vi "PDF_Interface_PDF Protokoll Dichtheitstest.vi"(8 "error in (no error)":errorcluster caption="Fehler (Eingang, kein Fehler)", 11 "Save PDF File Path":path) -> (0 "error out":errorcluster caption="Fehler (Ausgang)")   [LabVIEW 2020, in "Erweiterte Konfig.lvlib"]
uses:
  Erweiterte Konfig.lvlib
  Dichtheitstest Umfang.ctl
  Sprachverwaltung/FGV Aktion Tabelle zerlegen.ctl
  System Einstellungen V2/Aktioen FGV System Konstanten.ctl
  Status Dichtheitstest Aktionen.ctl
  FGV PID Aktionen.ctl
  PDF_Interface/PDF Protokoll Standard Kopf Optionen.ctl
  <vilib>/Simplicity AI/SAI_PDF_API/Classes/Context/Controls/SAI_PDF_PDF Details.ctl
  PDF_Interface/PDF Interface Helper/PDFContentType.ctl
  PDF_Interface/PDF Interface Helper/PDFTableContentType.ctl
  PDF_Interface/PDF Interface Helper/PDFResults.ctl
  PDF_Interface/PDF Interface Helper/PDFResultPictures.ctl
  PDF_Interface/PDF Interface Helper/PDFCommentPosition.ctl
  PDF_Interface/PDF Interface Helper/PDFPageBreak.ctl
  PDF_Interface/PDF Interface Helper/PDFTablePictures.ctl
  PDF_Interface/PDF Interface Helper/PDFBemerkung.ctl
  <vilib>/Simplicity AI/SAI_PDF_API/Classes/Context/Controls/SAI_PDF_Text Align.ctl
  <vilib>/Simplicity AI/SAI_PDF_API/Classes/Context/Controls/SAI_PDF_Font.ctl
  <vilib>/Simplicity AI/SAI_PDF_API/Classes/Context/Controls/SAI_PDF_Font Encoding.ctl
  Allgemein/allgemeine Sub-VIs.lvlib
  System Einstellungen V2/System Einstellungen V2.lvlib
  Sprachverwaltung/Sprachverwaltung.lvlib
  PDF_Interface/PDF Interface.lvlib
  <vilib>/Simplicity AI/SAI_PDF_API/Classes/Context/Context.lvclass
  PDF_Interface/PDF Interface Helper/PDF Interface Helper.lvlib
  Linearisierung V2/Protokoll/Protokoll.lvlib
panel:
  out "Dichtheitstest Umfang":T1 items=["Pumpe / Filter / FT-IR / PNS", "Pumpe / Filter / FT-IR", "Filter / FT-IR", "FT-IR"]
  out "zul. Druckabfall:":string
  out "Dauer Dichtheitstest:":string
  out "Bestanden":bool caption="Boolesch"
  out "Druckanstieg:":string
  out "Enddruck:":string
  out "Startdruck:":string
  out "Umfang:":string
  out "Endzeit:":string
  out "Startzeit:":string
  out "Ser.Nr.:":string caption="Serien Nummer:"
  out "Messgerät:":string
  # "Dichtheitstest"
  # "mbar"
  # "mbar"
  # "mbar"
  # "IAG-Industrie Automatisierungsgeschellschaft m.b.H.    l  Industriestraße 2    l    2722Weikersdorf     )+43262221734 7+43262221734655"
  # "mbar"
  # "s"
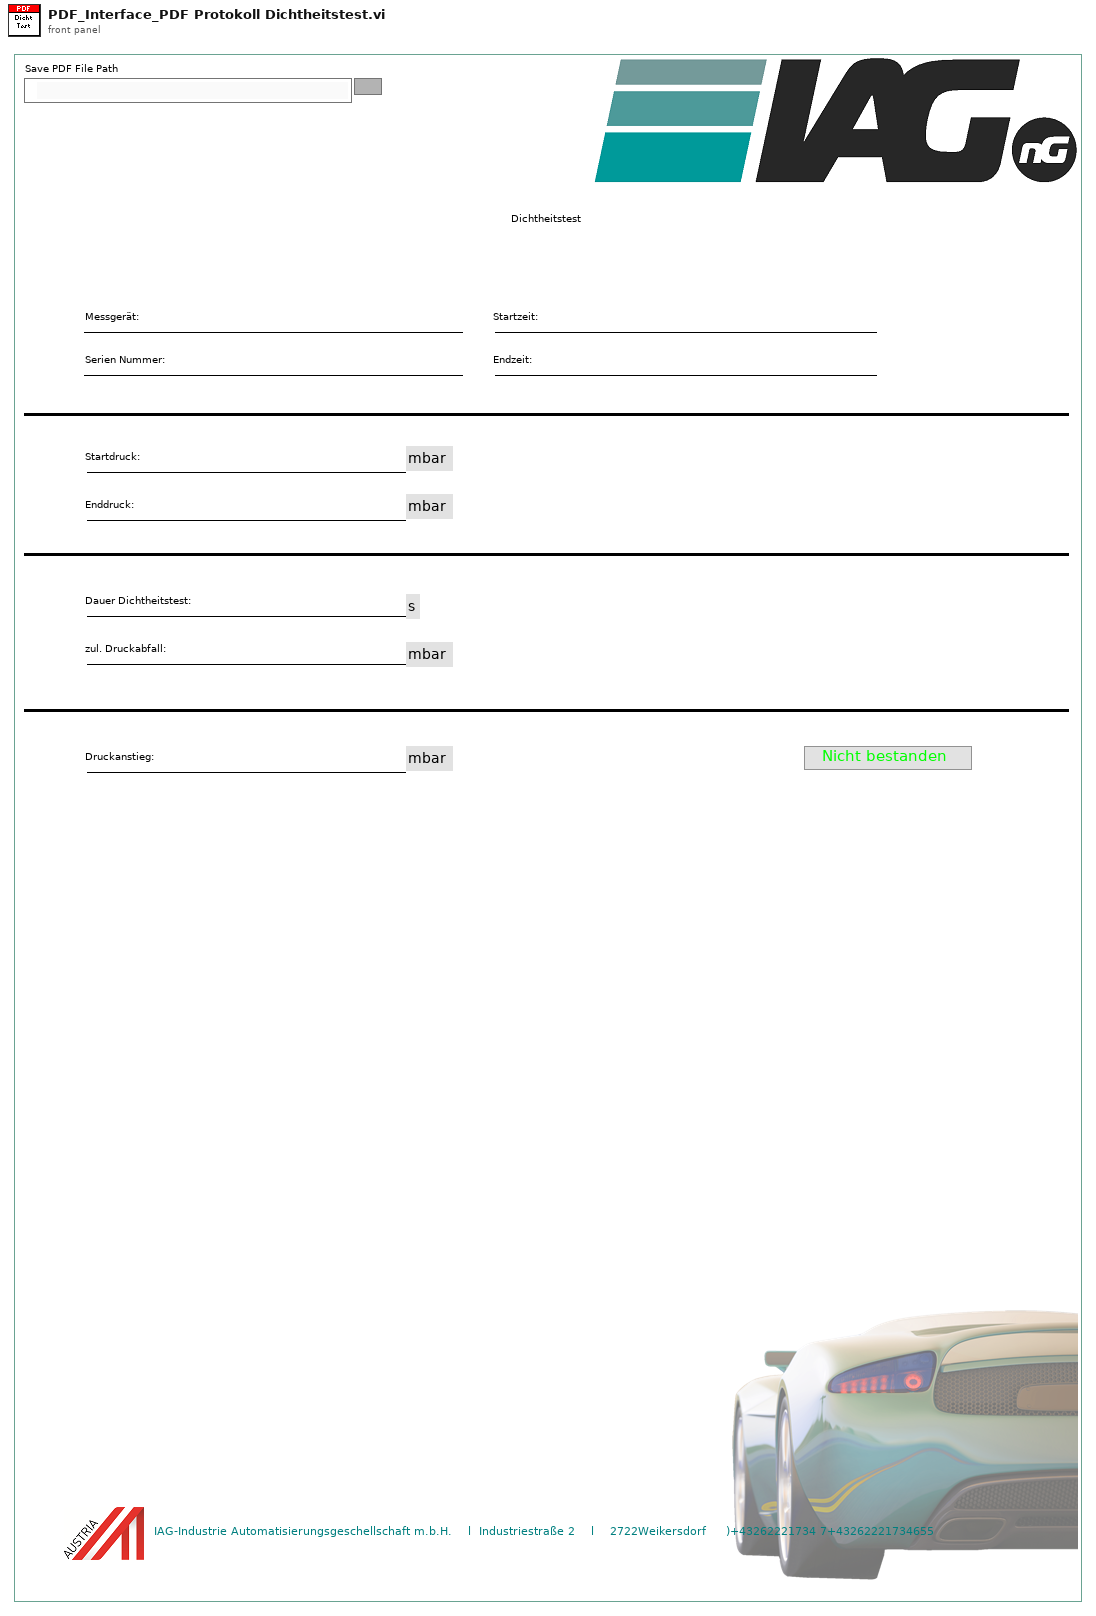
[diagram p1: front panel]
types:
  T1 = typedef "Erweiterte Konfig.lvlib/Dichtheitstest Umfang.ctl" = u16
  T2 = typedef "Sprachverwaltung.lvlib/FGV Aktion Tabelle zerlegen.ctl" = enum16{"laden", "vereinzeln", "speichern"}
  T3 = typedef "PDF Interface.lvlib/PDF Protokoll Standard Kopf Optionen.ctl" = cluster{"Analysator":bool, "FT-IR Rezept":bool, "Gasteiler":bool, "Gas Komponente":bool, "Gas Flasche":bool, "LIN Protokoll":bool, "Operator":bool}
  T4 = typedef "Erweiterte Konfig.lvlib/FGV PID Aktionen.ctl" = enum16{"Lesen", "Schreiben PID", "Schreiben Sonstige", "Dichtheitstest", "Aktionen Dicht.", "Parameter Sensor"}
  T5 = typedef "Erweiterte Konfig.lvlib/Status Dichtheitstest Aktionen.ctl" = enum16{"lesen", "Zeitstempel", "Daten", "läuft", "Protokolldaten"}
  T6 = typedef "System Einstellungen V2.lvlib/Aktioen FGV System Konstanten.ctl" = enum16{"lesen", "laden", "speichern", "Sprache"}
  T7 = typedef "PDF Interface.lvlib/PDF Interface Helper.lvlib/PDFBemerkung.ctl" = cluster{"Bemerkung Text":string, "Align (Left)":T8, "Add Line Feeds (F:No)":bool, "Font":T9}
  T8 = typedef "SAI_PDF_Toolkit.lvlib/Context.lvclass/SAI_PDF_Text Align.ctl" = i32
  T9 = typedef "SAI_PDF_Toolkit.lvlib/Context.lvclass/SAI_PDF_Font.ctl" = cluster{"Font":string, "Size":i32, "Colour":u32, "Bold":bool, "Italic":bool, "Underline":bool, "Strikethrough":bool, "Font Encoding":T10}
  T10 = typedef "SAI_PDF_Toolkit.lvlib/Context.lvclass/SAI_PDF_Font Encoding.ctl" = enum16{"Cp1252, WinANSI", "IdentityH", "IdentityV", "Cp1250", "Cp1257", "MacRoman"}
  T11 = typedef "PDF Interface.lvlib/PDF Interface Helper.lvlib/PDFResults.ctl" = cluster{"Results":cluster{"Result Text":string, "Result":bool}[], "ResultPictures":T12, "use Pictures":bool, "Image Scale (%)":sgl, "Autoscale? (T)":bool, "Horizontal Align":i32, "Position":i32}
  T12 = typedef "PDF Interface.lvlib/PDF Interface Helper.lvlib/PDFResultPictures.ctl" = cluster{"Yes Ctl Refnum":refnum<vi>, "No Ctl Refnum":refnum<vi>}
  T13 = typedef "PDF Interface.lvlib/PDF Interface Helper.lvlib/PDFTableContentType.ctl" = cluster{"TableHeader":string[], "Table":string[][], "Relative Column Widths (%)":sgl[], "Results":T11, "PositionBemerkung":T14, "PageBreak":T15, "TablePictures":T16, "Horizontal Align":i32}
  T14 = typedef "PDF Interface.lvlib/PDF Interface Helper.lvlib/PDFCommentPosition.ctl" = enum16{"before", "after"}
  T15 = typedef "PDF Interface.lvlib/PDF Interface Helper.lvlib/PDFPageBreak.ctl" = enum16{"none", "before", "after", "after comment"}
  T16 = typedef "PDF Interface.lvlib/PDF Interface Helper.lvlib/PDFTablePictures.ctl" = cluster{"Ctl Refnum In":refnum<vi>[], "RowOrColumn":enum16{"Row", "Column"}, "IndexToInsert":u16, "Image Scale (%)":sgl[], "Autoscale? (T)":bool[], "Horizontal Align":i32}
  T17 = typedef "PDF Interface.lvlib/PDF Interface Helper.lvlib/PDFContentType.ctl" = cluster{"Titel":string, "Header Table":string[][], "Table Array":T13[], "Bemerkungen":T7[]}
  T18 = typedef "SAI_PDF_Toolkit.lvlib/Context.lvclass/SAI_PDF_PDF Details.ctl" = cluster{"Title":string, "Subject":string, "Keywords":string, "Author":string, "Creator":string}
  T19 = cluster{"Header Footer Text Cluster":cluster{"Header Text":string, "Footer Text":string, "Time":string, "Page Number":string}, "PDF Details":T18}
  T20 = typedef "Erweiterte Konfig.lvlib/Dichtheitstest Protokoll.ctl" = cluster{"Startzeit":timestamp, "Endzeit":timestamp, "Startdruck":sgl, "Enddruck":sgl, "Dichtheitstest Umfang":T1}
  T21 = typedef "Erweiterte Konfig.lvlib/Sonstige Parameter.ctl" = cluster{"Lüfter langsam":sgl, "Lüfter schnell":sgl, "FT-IR Kühlung Soll":sgl, "FT-IR Kühlung Max":sgl, "Überwachung":T22, "Befüllung aktiv":T23, "Stickstoff Befüllzeit":sgl, "Befüllintervall":sgl, "Kalibrierwert FT-IR":sgl, "Offset Ausgang":sgl, "Offset FT-IR":sgl, "Offset Druck FT-IR":sgl, "Dichtheitstest Zeit":sgl, "Dichtheitstest Abfall":sgl, "Dichtheitstest Umfang":T1, "Offset Umgebung":sgl, "Max Taupunkt":sgl, "Pumpendrehzahl":sgl, "ext. Befüllung":T23, "Ext. Stickstoff Befüllzeit":sgl}
  T22 = typedef "Auswahlfeld.ctl" = u16
  T23 = typedef "LogKonfig.lvlib/Auswahlfeld aktiviert-deaktiviert.ctl" = u16
  T24 = cluster{"Header Size":i32, "Column Ratio left":sgl[]}
  T25 = typedef "String - Ausgabefeld.ctl" = string
  T26 = cluster{"Modell":string, "ProjektNummer":string, "Software Version":string, "Seriennummer":string}
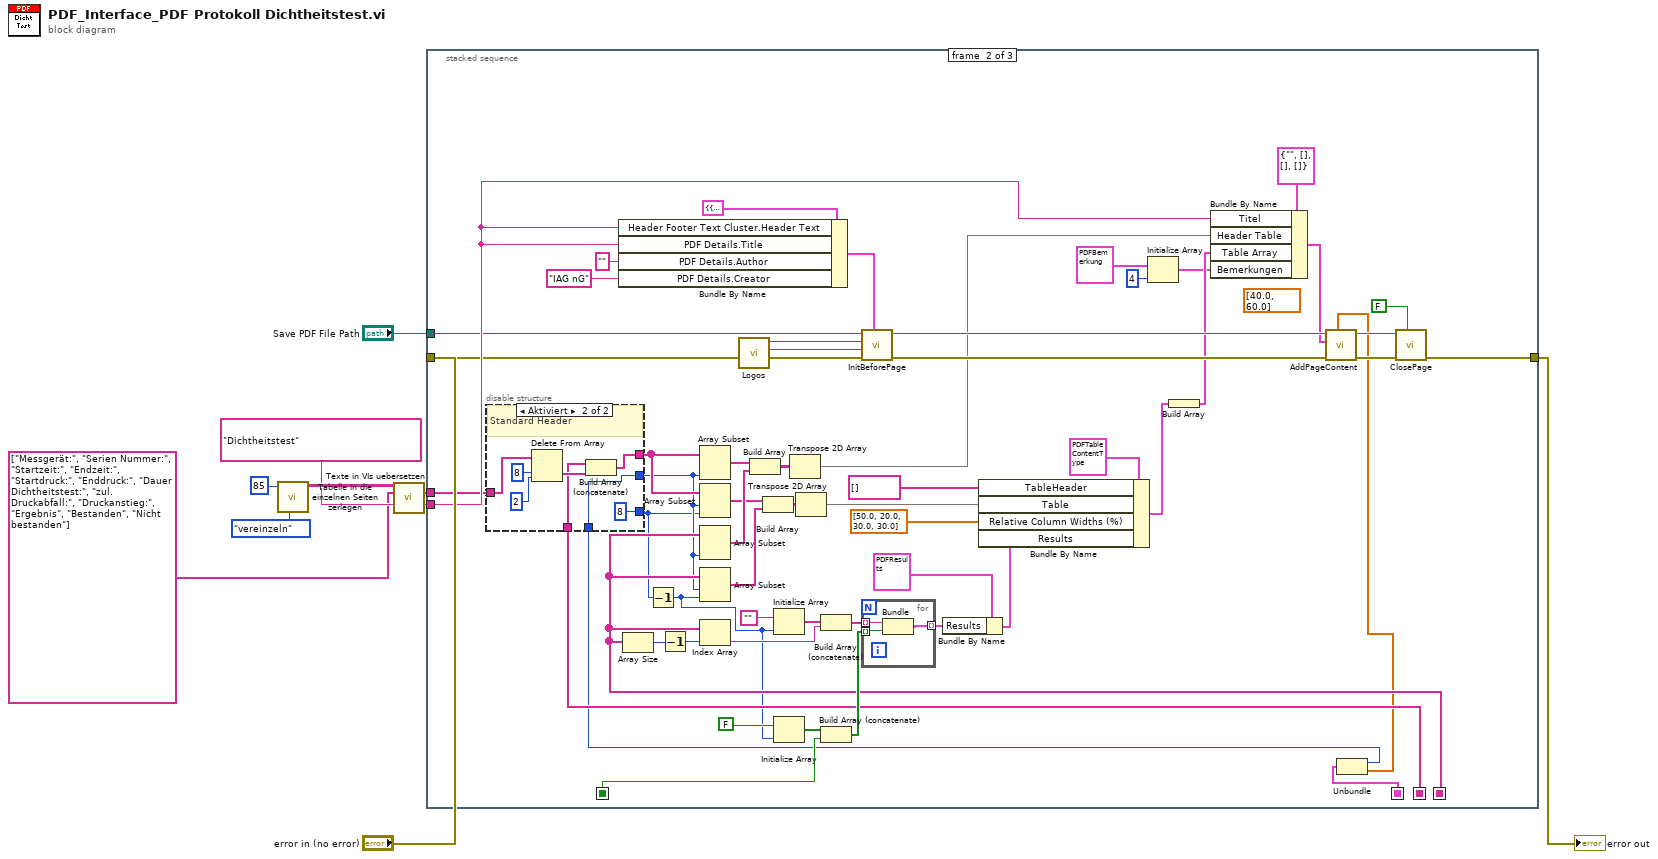
[diagram p0: block diagram]
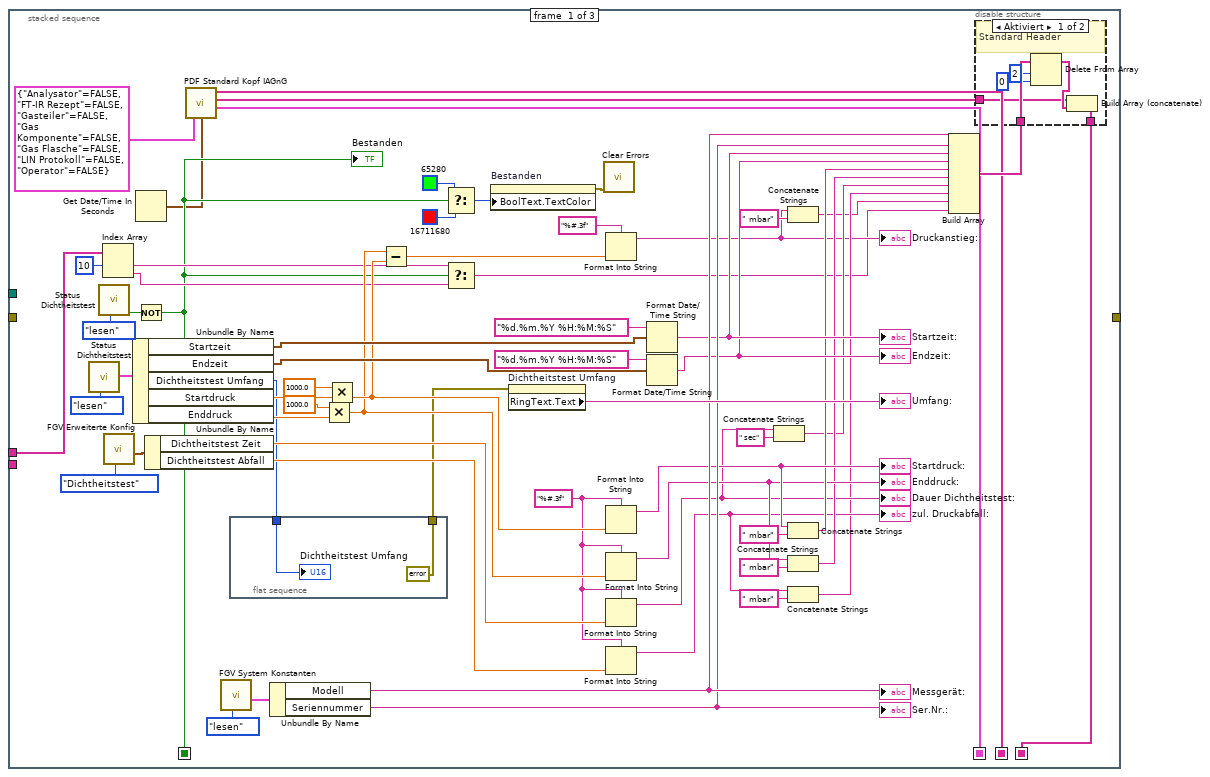
[diagram p2: hidden frame]
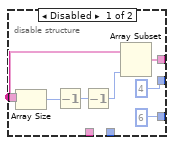
[diagram p4: hidden frame]
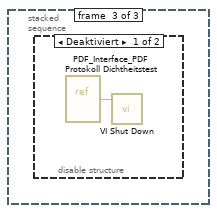
[diagram p5: hidden frame]
diagram:
  n1 = call "Tabelle in die einzelnen Seiten zerlegen.vi"("Aktion"=FGV_Aktion_Tabelle_zerlegen."vereinzeln", "Index (Seite)"=85) -> ("Sprachliste"=w8:string[][])  [unwired: 7 in, 2 out]
  n2 = call "Texte in VIs uebersetzen.vi"("Sprachliste"=w8, "String-Array zum Übersetzen"=string[] ["Messgerät:", "Serien Nummer:", "Startzeit:", "Endzeit:", "Startdruck:", "Enddruck:", "Dauer Dichtheitstest:", "zul. Druckabfall:", "Druckanstieg:", "Ergebnis", "Bestanden", "Nicht bestanden"], "String zum Übersetzen"="Dichtheitstest") -> ("String-Array zum Übersetzen"=w4:string[], "String zum Übersetzen"=w5:string)  [unwired: 8 in, 3 out]
  n3 = stacked-sequence {
    seq-local: [w15 _ _] -> [_ w95 _]
    seq-local: [w18 _ _] -> [_ w94 _]
    seq-local: [w11 _ _] -> [_ w88 _]
    seq-local: [w13 _ _] -> [_ w84 _]
    tunnel: w5 -> [_ w100 _]
    tunnel: w4 -> [w22 w99 _]
    tunnel: "Save PDF File Path" -> [_ w98 _]
    tunnel: "error in (no error)" -> [_ w97 _]
    tunnel: [_ w96 _] -> w1
    frame #0 {
      w46 = "%#.3f" ("Format-String")
      n4 = call "Status Dichtheitstest.vi"("Aktionen"=Status_Dichtheitstest_Aktionen."lesen") -> ("Protokoll"=w61:T20)  [unwired: 6 in, 4 out]
      n5 = call "Status Dichtheitstest.vi"("Aktionen"=Status_Dichtheitstest_Aktionen."lesen") -> ("Fehler"=w54:bool)  [unwired: 6 in, 4 out]
      n6 = Index Array(array=w22, index #1=10 ("Index")) -> (element #1=w20:string, element #2=w19:string)  [unwired: 1 in]
      n7 = call "FGV Erweiterte Konfig.vi"("Aktion"=FGV_PID_Aktionen."Dichtheitstest") -> ("Sonstige"=w57:T21)  [unwired: 6 in, 4 out]
      n8 = Unbundle By Name(w61) -> ("Startzeit"=w60:timestamp, "Endzeit"=w59:timestamp, "Dichtheitstest Umfang"=w45:T1, "Startdruck"=w53:sgl, "Enddruck"=w52:sgl)
      n9 = Get Date/Time In Seconds() -> (seconds since 1Jan1904=w12:timestamp)
      n10 = Not(x=w54) -> (.not. x?=w18:bool)
      "Bestanden" <- w18
      n11 = Unbundle By Name(w57) -> ("Dichtheitstest Zeit"=w56:sgl, "Dichtheitstest Abfall"=w55:sgl)
      n12 = call "PDF Standard Kopf IAGnG.vi"("Zeitstempel"=w12, "Oprtionen Cluster"=T3 {"Analysator"=FALSE, "FT-IR Rezept"=FALSE, "Gasteiler"=FALSE, "Gas Komponente"=FALSE, "Gas Flasche"=FALSE, "LIN Protokoll"=FALSE, "Operator"=FALSE}) -> ("Size Cluster"=w13:T24, "Header Values"=w14:T25[], "Header Labels"=w11:string[])  [unwired: 6 in, 1 out]
      n13 = call "FGV System Konstanten.vi"("Aktionen"=Aktioen_FGV_System_Konstanten."lesen") -> ("Cluster out"=w71:T26)  [unwired: 6 in, 4 out]
      n14 = flat-sequence {
        tunnel: w45 -> [w81]
        tunnel: [errorcluster {"status"=FALSE, "code"=0, "source"=""} ("Fehler (Eingang, kein Fehler)")] -> w43
        frame #0 {
          "Dichtheitstest Umfang" <- w81
        }
      }
      n15 = Unbundle By Name(w71) -> ("Modell"=w42:string, "Seriennummer"=w41:string)
      "Messgerät:" <- w42
      "Ser.Nr.:" <- w41
      n16 = Multiply(x=sgl 1000.0, y=w52) -> (x*y=w49:sgl)
      n17 = Multiply(x=sgl 1000.0, y=w53) -> (x*y=w50:sgl)
      n18 = Subtract(x=w49, y=w50) -> (x-y=w51:sgl)
      n19 = Select(t=u32 65280, s=w18, f=u32 16711680) -> (s? t:f=w65:u32)
      n20 = Select(t=w20, s=w18, f=w19) -> (s? t:f=w23:string)
      n21 = property on="Bestanden" class="Bool. (strikt)"("BoolText.TextColor"=w65) -> (error out=w64:errorcluster)  [unwired: 2 in, 1 out]
      n22 = property on="Dichtheitstest Umfang" class="Ring (strikt)"(error in=w43) -> ("RingText.Text"=→"Umfang:":string)  [unwired: 1 in, 2 out]
      n23 = call <vilib>:"Clear Errors.vi"("error in (no error)"=w64) -> ()  [unwired: 5 in, 2 out]
      n24 = Format Into String(format string="%#.3f" ("Format-String"), w51) -> (resulting string=w25:string)  [unwired: 2 in, 1 out]
      "Druckanstieg:" <- w25
      n25 = Format Into String(format string=w46, w50) -> (resulting string=w33:string)  [unwired: 2 in, 1 out]
      "Startdruck:" <- w33
      n26 = Format Into String(format string=w46, w49) -> (resulting string=w31:string)  [unwired: 2 in, 1 out]
      "Enddruck:" <- w31
      n27 = Format Into String(format string=w46, w56) -> (resulting string=w29:string)  [unwired: 2 in, 1 out]
      "Dauer Dichtheitstest:" <- w29
      n28 = Format Into String(format string=w46, w55) -> (resulting string=w27:string)  [unwired: 2 in, 1 out]
      "zul. Druckabfall:" <- w27
      n29 = Format Date/Time String(time format string (%c)="%d.%m.%Y %H:%M:%S" ("Zeitformatierungs-String (%c)"), seconds (now)=w60) -> (date/time string=w40:string)  [unwired: 1 in]
      "Startzeit:" <- w40
      n30 = Format Date/Time String(time format string (%c)="%d.%m.%Y %H:%M:%S" ("Zeitformatierungs-String (%c)"), seconds (now)=w59) -> (date/time string=w39:string)  [unwired: 1 in]
      "Endzeit:" <- w39
      n31 = Concatenate Strings(w29, " sec" ("String")) -> (w28:string)
      n32 = Concatenate Strings(w25, " mbar" ("String")) -> (w24:string)
      n33 = Concatenate Strings(w33, " mbar" ("String")) -> (w32:string)
      n34 = Concatenate Strings(w31, " mbar" ("String")) -> (w30:string)
      n35 = Concatenate Strings(w27, " mbar" ("String")) -> (w26:string)
      n36 = Build Array(w42, w41, w40, w39, w32, w30, w28, w26, w24, w23) -> (w16:string[])
      n37 = disable-structure shown="Aktiviert" {
        disable-tunnel: w16 -> [w78 w79]
        disable-tunnel: [w74 w79] -> w15
        disable-tunnel: w14 -> [w73 _]
        frame Enabled {
          # "Standard Header"
          n38 = Delete From Array(array=w78, length=2 ("Länge"), index=0 ("Index")) -> (array with subset deleted=w75:string[])  [unwired: 1 out]
          n39 = Build Array (concatenate)(w73, w75) -> (w74:T25[])
        }
        frame Disabled {
        }
      }
    }
    frame #1 {
      (unwired) sgl[] [40.0, 60.0] ("Column Ratio left")
      n40 = Bundle By Name(cluster=T19 {"Header Footer Text Cluster"={"Header Text"="Protokoll XYZ", "Footer Text"="IAG nG", "Time"="<TIMESTAMP yyyy-MM-dd>", "Page Number"="Page <P> of <PT>"}, "PDF Details"={"Title"="Test PDF", "Subject"="Versa Tabasco", "Keywords"="", "Author"="RIW", "Creator"="IAG"}} ("Info"), "Header Footer Text Cluster.Header Text"=w100, "PDF Details.Title"=w100, "PDF Details.Author"="", "PDF Details.Creator"="IAG nG") -> (w127:T19)
      n41 = Array Size(array=w95) -> (size(s)=w121:i32)
      n42 = Decrement(x=w121) -> (x-1=w113:i32)
      n43 = Index Array(array=w95, index=w113) -> (element=w118:T25)
      n44 = call "Logos.vi"() -> ("Footer Image File Path"=w136:path, "Header Image File Path"=w137:path)  [unwired: 8 in, 2 out]
      n45 = call "InitBeforePage.vi"("Info"=w127, "Fehler (Eingang, kein Fehler)"=w97, "Footer Image File Path"=w136, "Header Image File Path"=w137, "Path (Dialog if Empty)"=w98) -> ("Fehler (Ausgang)"=w135:errorcluster, "Context (Ausgang)"=w134:refnum<class "Context.lvclass">)  [unwired: 5 in]
      n46 = Initialize Array(T7 {"Bemerkung Text"="", "Align (Left)"=0, "Add Line Feeds (F:No)"=FALSE, "Font"={"Font"="Arial", "Size"=10, "Colour"=0, "Bold"=FALSE, "Italic"=FALSE, "Underline"=FALSE, "Strikethrough"=FALSE, "Font Encoding"=enum."Cp1252, WinANSI"}} ("Bemerkung"), 4 ("Dimensionsgröße")) -> (w101:T7[])
      n47 = Unbundle(w84) -> ("Header Size"=w83:i32, "Column Ratio left"=w82:sgl[])
      n48 = disable-structure shown="Aktiviert" {
        disable-tunnel: [w141 w147] -> w122
        disable-tunnel: w99 -> [w140 w152]
        disable-tunnel: w88 -> [_ w148]
        disable-tunnel: [4 ("Länge") w146] -> w87
        disable-tunnel: [6 ("Länge") 8 ("Länge")] -> w86
        disable-tunnel: w83 -> [_ w146]
        frame Disabled {
          n49 = Array Size(array=w140) -> (size(s)=w144:i32)
          n50 = Decrement(x=w144) -> (x-1=w143:i32)
          n51 = Decrement(x=w143) -> (x-1=w142:i32)
          n52 = Array Subset(array=w140, length=w142) -> (w141:string[])  [unwired: 1 in]
        }
        frame Enabled {
          # "Standard Header"
          n53 = Delete From Array(array=w152, length=8 ("Länge"), index=2 ("Index")) -> (deleted portion=w149:string[])  [unwired: 1 out]
          n54 = Build Array (concatenate)(w148, w149) -> (w147:string[])
        }
      }
      n55 = Decrement(x=w86) -> (x-1=w85:i32)
      n56 = Array Subset(array=w122, length=w87) -> (w125:string[])  [unwired: 1 in]
      n57 = Array Subset(array=w122, index=w87, length=w86) -> (w116:string[])
      n58 = Array Subset(array=w95, length=w87) -> (w124:T25[])  [unwired: 1 in]
      n59 = Array Subset(array=w95, index=w87, length=w85) -> (w115:T25[])
      n60 = Build Array(w125, w124) -> (w123:T25[][])
      n61 = Build Array(w116, w115) -> (w114:T25[][])
      n62 = Initialize Array("", w85) -> (w119:string[])
      n63 = Initialize Array(FALSE, w85) -> (w111:bool[])
      n64 = Transpose 2D Array(2D array=w123) -> (transposed array=w104:T25[][])
      n65 = Transpose 2D Array(2D array=w114) -> (transposed array=w103:T25[][])
      n66 = Build Array (concatenate)(w119, w118) -> (w110:T25[])
      n67 = Build Array (concatenate)(w111, w94) -> (w109:bool[])
      n68 = for {
        tunnel: w110 -> [w155] mode=indexing
        tunnel: w109 -> [w154] mode=indexing
        tunnel: [w153] -> w92 mode=indexing
        n69 = Bundle("String - Ausgabefeld"=w155, w154) -> (w153:cluster{"String - Ausgabefeld":T25, bool})  [unwired: 1 in]
      }
      n70 = Bundle By Name(cluster=T11 {"Results"=[], "ResultPictures"={"Yes Ctl Refnum"=refnum, "No Ctl Refnum"=refnum}, "use Pictures"=FALSE, "Image Scale (%)"=100.0, "Autoscale? (T)"=TRUE, "Horizontal Align"=3, "Position"=0} ("Results"), "Results"=w92) -> (w90:T11)
      n71 = Bundle By Name(cluster=T13 {"TableHeader"=[], "Table"=[], "Relative Column Widths (%)"=[], "Results"={"Results"=[], "ResultPictures"={"Yes Ctl Refnum"=refnum, "No Ctl Refnum"=refnum}, "use Pictures"=FALSE, "Image Scale (%)"=0.0, "Autoscale? (T)"=FALSE, "Horizontal Align"=0, "Position"=0}, "PositionBemerkung"=enum."before", "PageBreak"=enum."none", "TablePictures"={"Ctl Refnum In"=[], "RowOrColumn"=enum."Row", "IndexToInsert"=0, "Image Scale (%)"=[], "Autoscale? (T)"=[], "Horizontal Align"=0}, "Horizontal Align"=0} ("Table Array"), "TableHeader"=string[] [], "Table"=w103, "Relative Column Widths (%)"=sgl[] [50.0, 20.0, 30.0, 30.0], "Results"=w90) -> (w107:T13)
      n72 = Build Array(w107) -> (w106:T13[])
      n73 = Bundle By Name(cluster=T17 {"Titel"="", "Header Table"=[], "Table Array"=[], "Bemerkungen"=[]} ("Content"), "Titel"=w100, "Header Table"=w104, "Table Array"=w106, "Bemerkungen"=w101) -> (w105:T17)
      n74 = call "AddPageContent.vi"("Column Ratio left"=w82, "error in"=w135, "Content"=w105, "Context (Eingang)"=w134) -> ("error out"=w133:errorcluster, "Context (Ausgang)"=w132:refnum<class "Context.lvclass">)  [unwired: 6 in]
      n75 = call "ClosePage.vi"("popup viewer"=FALSE, "Fehler (Eingang, kein Fehler)"=w133, "Context (Eingang)"=w132) -> ("Fehler (Ausgang)"=w96:errorcluster)  [unwired: 8 in]
    }
    frame #2 {
      n76 = disable-structure shown="Deaktiviert" {
        frame Disabled {
          n77 = vi-ref "PDF_Interface_PDF Protokoll Dichtheitstest.vi"() -> (w156:refnum<vi>)
          n78 = call "VI Shut Down.vi"("VI Referenz"=w156) -> ()  [unwired: 11 in]
        }
        frame Enabled {
        }
      }
    }
  }
  "error out" <- w1
